vi "Get Hand Profit or Loss.vi"(10 "Hand History String":string, 11 "Dealt Player Name":string) -> (3 "Profit/Loss":dbl)   [LabVIEW 2020]
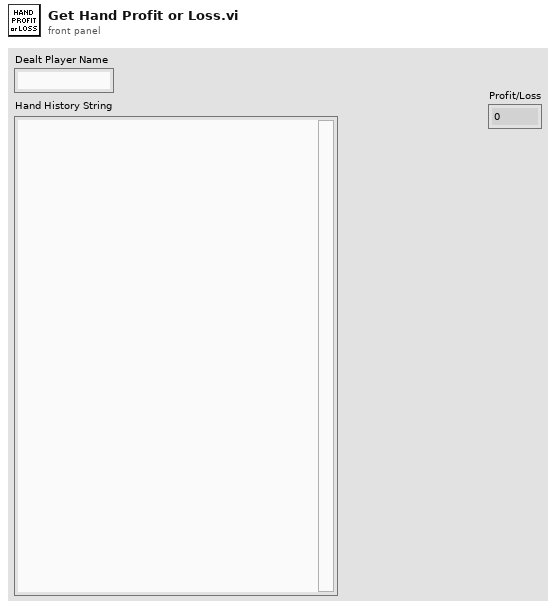
[diagram p1: front panel]
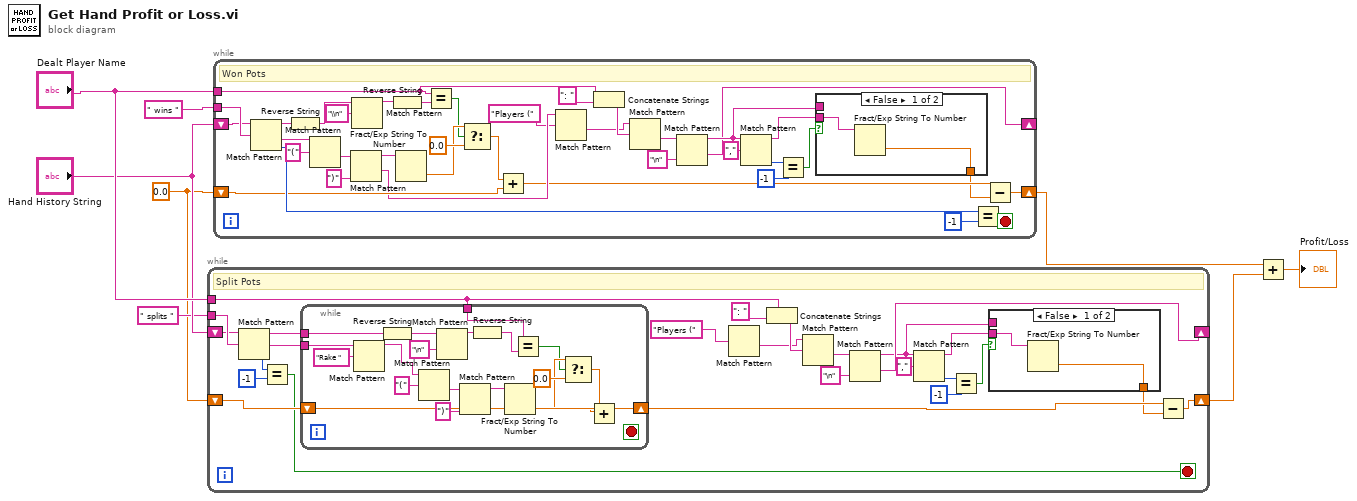
[diagram p0: block diagram]
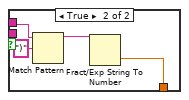
[diagram p2: hidden frame]
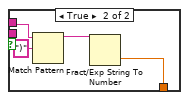
[diagram p3: hidden frame]
diagram:
  w1 = 0.0
  n1 = while {
    shift-right: [w27] -> _
    shift-left: "Hand History String" -> [w32]
    tunnel: " splits " ("string") -> [w33]
    tunnel: "Dealt Player Name" -> [w30]
    shift-right: [w29] -> w3
    shift-left: w1 -> [w31]
    stop <- w10 stop-if-true
    # "Split Pots"
    n2 = Match Pattern(string=w32, regular expression=w33) -> (before substring=w13:string, after substring=w9:string, offset past match=w11:i32)  [unwired: 1 in, 1 out]
    n3 = Equal?(x=w11, y=-1) -> (x = y?=w10:bool)
    n4 = while {
      tunnel: w30 -> [w51]
      tunnel: w13 -> [w49]
      tunnel: w9 -> [w47]
      shift-right: [w50] -> w28
      shift-left: w31 -> [w52]
      stop <- _ stop-if-true
      n5 = Match Pattern(string=w47, regular expression="Rake ") -> (before substring=w48:string)  [unwired: 1 in, 3 out]
      n6 = Reverse String(1:w49) -> (0:w42:string)
      n7 = Match Pattern(string=w48, regular expression="(") -> (after substring=w40:string)  [unwired: 1 in, 3 out]
      n8 = Match Pattern(string=w42, regular expression="\n") -> (before substring=w44:string)  [unwired: 1 in, 3 out]
      n9 = Match Pattern(string=w40, regular expression=")") -> (before substring=w38:string)  [unwired: 1 in, 3 out]
      n10 = Reverse String(1:w44) -> (0:w43:string)
      n11 = Fract/Exp String To Number(string=w38) -> (number=w36:dbl)  [unwired: 3 in, 1 out]
      n12 = Equal?(x=w51, y=w43) -> (x = y?=w35:bool)
      n13 = Select(t=w36, s=w35, f=0.0) -> (s? t:f=w34:dbl)
      n14 = Add(x=w34, y=w52) -> (x+y=w50:dbl)
    }
    n15 = Match Pattern(regular expression="Players (") -> (after substring=w23:string)  [unwired: 2 in, 3 out]
    n16 = Concatenate Strings(w30, ": " ("string")) -> (w24:string)
    n17 = Match Pattern(string=w23, regular expression=w24) -> (after substring=w16:string)  [unwired: 1 in, 3 out]
    n18 = Match Pattern(string=w16, regular expression="\n") -> (before substring=w14:string, after substring=w27:string)  [unwired: 1 in, 2 out]
    n19 = Match Pattern(string=w14, regular expression=",") -> (before substring=w18:string, offset past match=w21:i32)  [unwired: 1 in, 2 out]
    n20 = Equal?(x=w21, y=-1) -> (x = y?=w19:bool)
    n21 = case shown="False" w19 {
      tunnel: w18 -> [w54 _]
      tunnel: [w53 w55] -> w17
      tunnel: w14 -> [_ w58]
      frame False {
        n22 = Fract/Exp String To Number(string=w54) -> (number=w53:dbl)  [unwired: 3 in, 1 out]
      }
      frame True {
        n23 = Match Pattern(string=w58, regular expression=")") -> (before substring=w56:string)  [unwired: 1 in, 3 out]
        n24 = Fract/Exp String To Number(string=w56) -> (number=w55:dbl)  [unwired: 3 in, 1 out]
      }
    }
    n25 = Subtract(x=w28, y=w17) -> (x-y=w29:dbl)
  }
  n26 = while {
    shift-right: [w59] -> _
    shift-left: "Hand History String" -> [w95]
    tunnel: " wins " ("string") -> [w96]
    tunnel: "Dealt Player Name" -> [w74]
    shift-right: [w70] -> w4
    shift-left: w1 -> [w81]
    stop <- w94 stop-if-true
    # "Won Pots"
    n27 = Match Pattern(string=w95, regular expression=w96) -> (before substring=w91:string, after substring=w86:string, offset past match=w93:i32)  [unwired: 1 in, 1 out]
    n28 = Reverse String(1:w91) -> (0:w87:string)
    n29 = Match Pattern(string=w86, regular expression="(") -> (after substring=w84:string)  [unwired: 1 in, 3 out]
    n30 = Match Pattern(string=w84, regular expression=")") -> (before substring=w82:string, after substring=w76:string)  [unwired: 1 in, 2 out]
    n31 = Match Pattern(string=w87, regular expression="\\n") -> (before substring=w89:string)  [unwired: 1 in, 3 out]
    n32 = Reverse String(1:w89) -> (0:w88:string)
    n33 = Fract/Exp String To Number(string=w82) -> (number=w79:dbl)  [unwired: 3 in, 1 out]
    n34 = Equal?(x=w74, y=w88) -> (x = y?=w78:bool)
    n35 = Select(t=w79, s=w78, f=0.0) -> (s? t:f=w77:dbl)
    n36 = Add(x=w77, y=w81) -> (x+y=w69:dbl)
    n37 = Match Pattern(string=w76, regular expression="Players (") -> (after substring=w71:string)  [unwired: 1 in, 3 out]
    n38 = Concatenate Strings(w74, ": " ("string")) -> (w72:string)
    n39 = Match Pattern(string=w71, regular expression=w72) -> (after substring=w62:string)  [unwired: 1 in, 3 out]
    n40 = Match Pattern(string=w62, regular expression="\n") -> (before substring=w60:string, after substring=w59:string)  [unwired: 1 in, 2 out]
    n41 = Match Pattern(string=w60, regular expression=",") -> (before substring=w64:string, offset past match=w67:i32)  [unwired: 1 in, 2 out]
    n42 = Equal?(x=w67, y=-1) -> (x = y?=w65:bool)
    n43 = case shown="False" w65 {
      tunnel: w64 -> [w98 _]
      tunnel: [w97 w99] -> w63
      tunnel: w60 -> [_ w102]
      frame False {
        n44 = Fract/Exp String To Number(string=w98) -> (number=w97:dbl)  [unwired: 3 in, 1 out]
      }
      frame True {
        n45 = Match Pattern(string=w102, regular expression=")") -> (before substring=w100:string)  [unwired: 1 in, 3 out]
        n46 = Fract/Exp String To Number(string=w100) -> (number=w99:dbl)  [unwired: 3 in, 1 out]
      }
    }
    n47 = Equal?(x=w93, y=-1) -> (x = y?=w94:bool)
    n48 = Subtract(x=w69, y=w63) -> (x-y=w70:dbl)
  }
  n49 = Add(x=w4, y=w3) -> (x+y=→"Profit/Loss":dbl)
